vi "detector-select.vi"(3 "Detector Select":u16(ring) items=["InGaAs"=1, "CCD"=0], 4 "Cooling Status":T2={"Newton Init"=FALSE, "Newton Cooling"=FALSE, "Newton Parameters "=FALSE, "iDus Init"=FALSE, "iDus Cooling"=FALSE, "iDus Parameters"=FALSE, "Clara Init"=FALSE, "Clara Cooling"=FALSE, "Clara Parameters"=FALSE, "Newton Cooler StatusCode"=enum."DRV_TEMPERATURE_NOT_SUPPORTED", "iDus Cooler StatusCode"=enum."DRV_TEMPERATURE_NOT_SUPPORTED", "Clara Cooler StatusCode"=enum."DRV_TEMPERATURE_NOT_SUPPORTED"}, 5 "Handle":cluster{"iDus":i32, "Newton":i32, "Clara":i32} caption="Handle Cluster") -> (0 "Current Detector":string, 1 "Current Handle":i32, 2 "Detector Status":bool)   [LabVIEW 2015]
uses:
  <userlib>/atmcd32d.llb/Error Code Enum typedef.ctl
panel:
  # "Init"
  # "Cooling"
  # "Parameters"
  # "Newton"
  # "iDus"
  # "Clara"
  # "Clara"
  # "iDus"
  # "Newton"
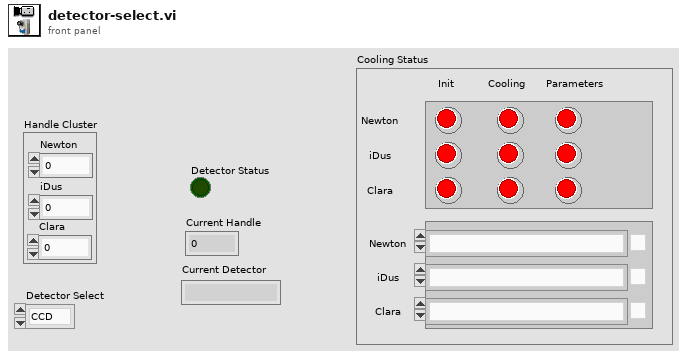
[diagram p1: front panel]
types:
  T1 = typedef "Error Code Enum typedef.ctl" = enum32{"N/A (0)", "DRV_ERROR_CODES", "DRV_SUCCESS", "DRV_VXDNOTINSTALLED", "DRV_ERROR_SCAN", "DRV_ERROR_CHECK_SUM", "DRV_ERROR_FILELOAD", "DRV_UNKNOWN_FUNC", "DRV_ERROR_VXD_INIT", "DRV_ERROR_ADDRESS", "DRV_ERROR_PAGELOCK", "DRV_ERROR_PAGEUNLOCK", "DRV_ERROR_BOARDTEST", "DRV_ERROR_ACK", "DRV_ERROR_UP_FIFO", "DRV_ERROR_PATTERN", "N/A (16)", "DRV_ACQUISITION_ERRORS", "DRV_ACQ_BUFFER", "DRV_ACQ_DOWNFIFO_FULL", "DRV_PROC_UNKONWN_INSTRUCTION", "DRV_ILLEGAL_OP_CODE", "DRV_KINETIC_TIME_NOT_MET", "DRV_ACCUM_TIME_NOT_MET", "DRV_NO_NEW_DATA", "N/A (25)", "DRV_SPOOLERROR", "N/A (27)", "N/A (28)", "N/A (29)", "N/A (30)", "N/A (31)", "N/A (32)", "DRV_TEMPERATURE_CODES", "DRV_TEMPERATURE_OFF", "DRV_TEMPERATURE_NOT_STABILIZED", "DRV_TEMPERATURE_STABILIZED", "DRV_TEMPERATURE_NOT_REACHED", "DRV_TEMPERATURE_OUT_RANGE", "DRV_TEMPERATURE_NOT_SUPPORTED", "DRV_TEMPERATURE_DRIFT", "N/A (41)", "N/A (42)", "N/A (43)", "N/A (44)", "N/A (45)", "N/A (46)", "N/A (47)", "N/A (48)", "DRV_GENERAL_ERRORS", "DRV_INVALID_AUX", "DRV_COF_NOTLOADED", "DRV_FPGAPROG", "DRV_FLEXERROR", "DRV_GPIBERROR", "N/A (55)", "N/A (56)", "N/A (57)", "N/A (58)", "N/A (59)", "N/A (60)", "N/A (61)", "N/A (62)", "N/A (63)", "DRV_DATATYPE", "DRV_DRIVER_ERRORS", "DRV_P1INVALID", "DRV_P2INVALID", "DRV_P3INVALID", "DRV_P4INVALID", "DRV_INIERROR", "DRV_COFERROR", "DRV_ACQUIRING", "DRV_IDLE", "DRV_TEMPCYCLE", "DRV_NOT_INITIALIZED", "DRV_P5INVALID", "DRV_P6INVALID", "DRV_INVALID_MODE", "DRV_INVALID_FILTER", "DRV_I2CERRORS", "DRV_I2CDEVNOTFOUND", "DRV_I2CTIMEOUT", "DRV_P7INVALID", "N/A (84)", "N/A (85)", "N/A (86)", "N/A (87)", "N/A (88)", "N/A (89)", "DRV_IOCERROR", "DRV_VRMVERSIONERROR"}
  T2 = cluster{"Newton Init":bool, "Newton Cooling":bool, "Newton Parameters ":bool, "iDus Init":bool, "iDus Cooling":bool, "iDus Parameters":bool, "Clara Init":bool, "Clara Cooling":bool, "Clara Parameters":bool, "Newton Cooler StatusCode":T1, "iDus Cooler StatusCode":T1, "Clara Cooler StatusCode":T1}
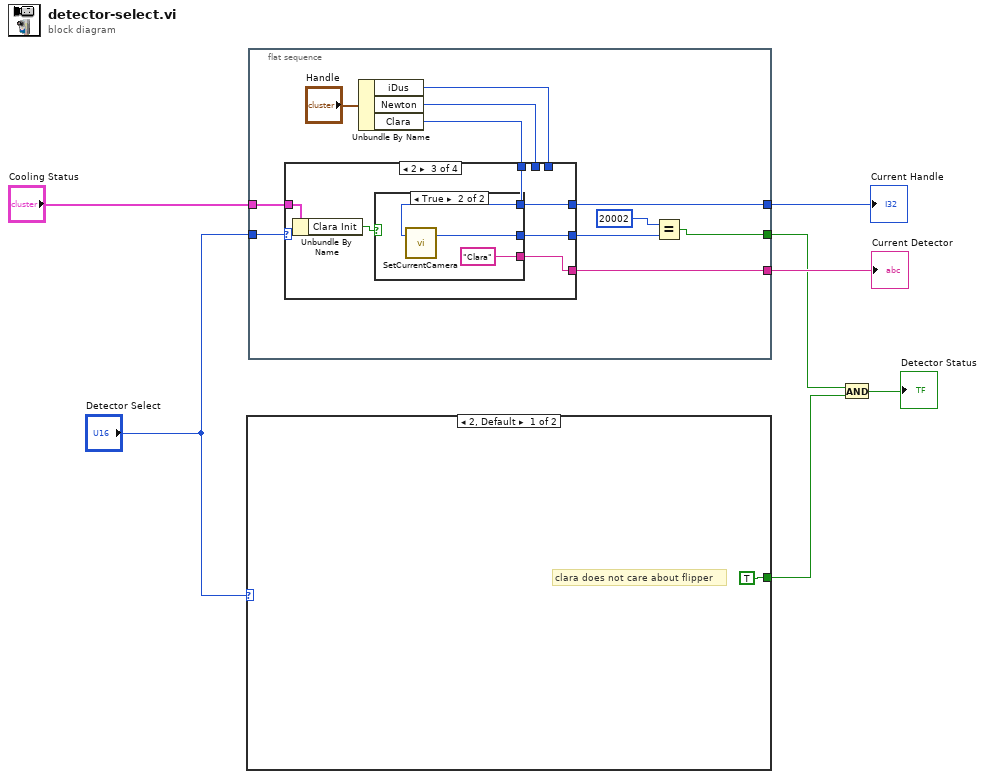
[diagram p0: block diagram]
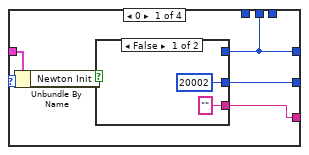
[diagram p2: hidden frame]
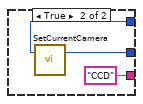
[diagram p3: hidden frame]
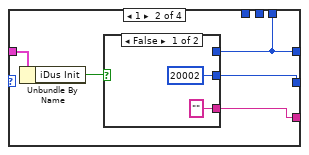
[diagram p4: hidden frame]
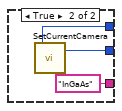
[diagram p5: hidden frame]
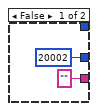
[diagram p6: hidden frame]
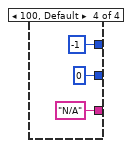
[diagram p7: hidden frame]
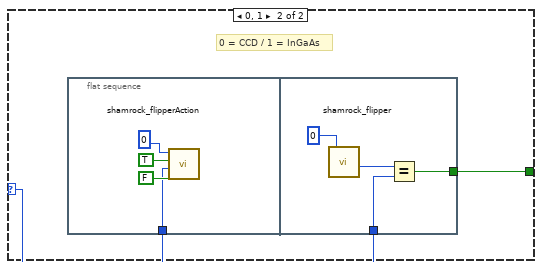
[diagram p8: hidden frame]
diagram:
  n1 = case shown="2, Default" "Detector Select" {
    selector: "Detector Select" -> [_ w10]
    tunnel: [TRUE w9] -> w4
    frame 2, Default {
      # "clara does not care about flipper"
    }
    frame 0, 1 {
      # "0 = CCD / 1 = InGaAs"
      n2 = flat-sequence {
        tunnel: w10 -> [w11]
        tunnel: w10 -> [w16]
        tunnel: [w15] -> w9
        frame #0 {
          n3 = call <userlib>:"shamrock_flipperAction.vi"("FlipperReset"=FALSE, "Port"=w11, "SetPort"=TRUE, "Device No"=0) -> ()  [unwired: 2 out]
        }
        frame #1 {
          n4 = call <userlib>:"shamrock_flipper.vi"("Device No"=0) -> ("Port"=w17:i32)  [unwired: 6 out]
          n5 = Equal?(x=w17, y=w16) -> (x = y?=w15:bool)
        }
      }
    }
  }
  n6 = flat-sequence {
    tunnel: [w29] -> w7
    tunnel: [w28] -> w6
    tunnel: "Detector Select" -> [w23]
    tunnel: [w20] -> w2
    tunnel: "Cooling Status" -> [w19]
    frame #0 {
      n7 = Unbundle By Name("Handle") -> ("iDus"=w25:i32, "Newton"=w26:i32, "Clara"=w27:i32)
      n8 = case shown="2" w23 {
        tunnel: w25 -> [_ w44 _ _]
        tunnel: w26 -> [w34 _ _ _]
        tunnel: [w32 w42 w52 "N/A"] -> w29
        tunnel: [w34 w44 w53 -1 ("Clara")] -> w28
        tunnel: [w33 w43 w54 u32 0 ("DLL error code")] -> w22
        tunnel: w27 -> [_ _ w53 _]
        tunnel: w19 -> [w31 w41 w51 _]
        frame 0 {
          n9 = Unbundle By Name(w31) -> ("Newton Init"=w30:bool)
          n10 = case shown="False" w30 {
            tunnel: w34 -> [_ w39]
            tunnel: [u32 20002 ("DLL error code") w38] -> w33
            tunnel: ["" "CCD"] -> w32
            frame False {
            }
            frame True {
              n11 = call <userlib>:"SetCurrentCamera.vi"("cameraHandle"=w39) -> ("DLL error code"=w38:u32)  [unwired: 1 in, 1 out]
            }
          }
        }
        frame 1 {
          n12 = Unbundle By Name(w41) -> ("iDus Init"=w40:bool)
          n13 = case shown="False" w40 {
            tunnel: w44 -> [_ w49]
            tunnel: [u32 20002 ("DLL error code") w48] -> w43
            tunnel: ["" "InGaAs"] -> w42
            frame False {
            }
            frame True {
              n14 = call <userlib>:"SetCurrentCamera.vi"("cameraHandle"=w49) -> ("DLL error code"=w48:u32)  [unwired: 1 in, 1 out]
            }
          }
        }
        frame 2 {
          n15 = Unbundle By Name(w51) -> ("Clara Init"=w50:bool)
          n16 = case shown="True" w50 {
            tunnel: [u32 20002 ("DLL error code") w59] -> w54
            tunnel: w53 -> [_ w58]
            tunnel: ["" "Clara"] -> w52
            frame False {
            }
            frame True {
              n17 = call <userlib>:"SetCurrentCamera.vi"("cameraHandle"=w58) -> ("DLL error code"=w59:u32)  [unwired: 1 in, 1 out]
            }
          }
        }
        frame 100, Default {
        }
      }
      n18 = Equal?(x=u32 20002 ("= temperature\naccepted"), y=w22) -> (x = y?=w20:bool)
    }
  }
  n19 = And(x=w2, y=w4) -> (x .and. y?=→"Detector Status":bool)
  "Current Detector" <- w7
  "Current Handle" <- w6
